vi "DAC TC Temperature FP Conf.vi"(6 "Used TC Temps":bool[](array[boolean]), 8 "error in (no error)":errorcluster, 9 "Active TC names":string, 10 "Result Unit":string, 11 "DeepU Results in":refnum<class "DeepU Results.lvclass">) -> (0 "error out":errorcluster, 3 "DeepU Results out":refnum<class "DeepU Results.lvclass">)   [LabVIEW 2019, in "Results.lvlib" / "DeepU Results.lvclass"]
uses:
  DeepU Results.lvclass
  DeepU Results.lvclass/DeepU Results.ctl
panel:
  out "size(s)":i32
  out "Array":bool[](array[boolean])
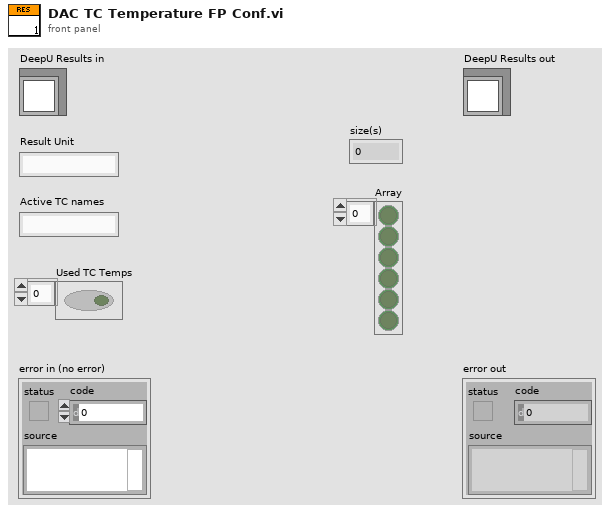
[diagram p1: front panel]
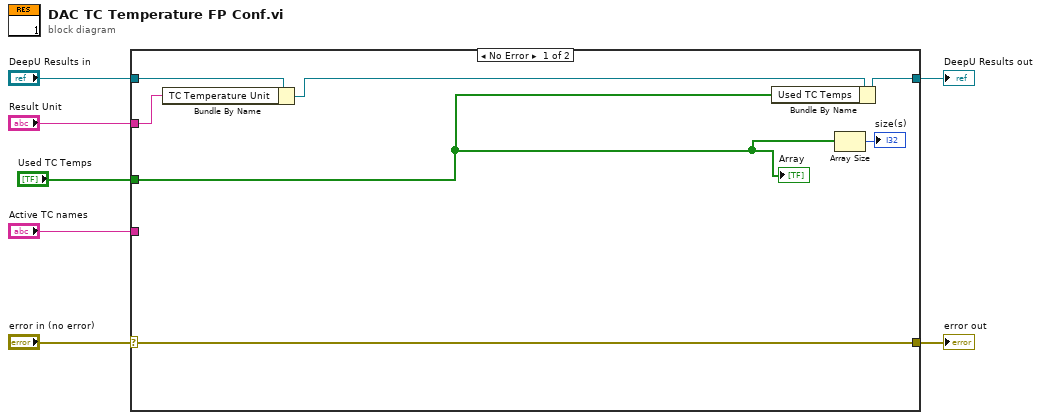
[diagram p0: block diagram]
diagram:
  n1 = case shown="No Error" "error in (no error)" {
    selector: "error in (no error)" -> [w14 w16]
    tunnel: [w14 w16] -> w6
    tunnel: [w10 w15] -> w4
    tunnel: "DeepU Results in" -> [w12 w15]
    tunnel: "Active TC names" -> [_ _]
    tunnel: "Result Unit" -> [w11 _]
    tunnel: "Used TC Temps" -> [w8 _]
    frame No Error {
      n2 = Bundle By Name(cluster=w12, "TC Temperature Unit"=w11) -> (w13:refnum<class "DeepU Results.lvclass">)
      n3 = Bundle By Name(cluster=w13, "Used TC Temps"=w8) -> (w10:refnum<class "DeepU Results.lvclass">)
      n4 = Array Size(array=w8) -> (size(s)=→"size(s)":i32)
      "Array" <- w8
    }
    frame Error {
    }
  }
  "error out" <- w6
  "DeepU Results out" <- w4
